vi "Choreo_Choreo_Globals.vi"() -> ()   [LabVIEW 2019, in "ChoreoLib.lvlib"]
doc: "Global variables for the Choreo Trajectory following system."
uses:
  ChoreoLib.lvlib
  TypeDef/ChoreoTrajectoryCacheSwerve.ctl
  TypeDef/ChoreoTrajectorySwerve.ctl
  TypeDef/ChoreoSwerveSample.ctl
  TypeDef/ChoreoEventMarker.ctl
  ENum/Choreo_Util_AllianceFlipType.ctl
panel:
  in  "AllianceFlipYearInfo":T2={"Year"=2026, "AllianceFlipType"=enum."ROTATE_AROUND", "FieldLength"=16.541, "FieldWidth"=8.0692}
  in  "TrajectoryCacheSwerve":T3
  # "NOTE: This will need to be updated\nevery year."
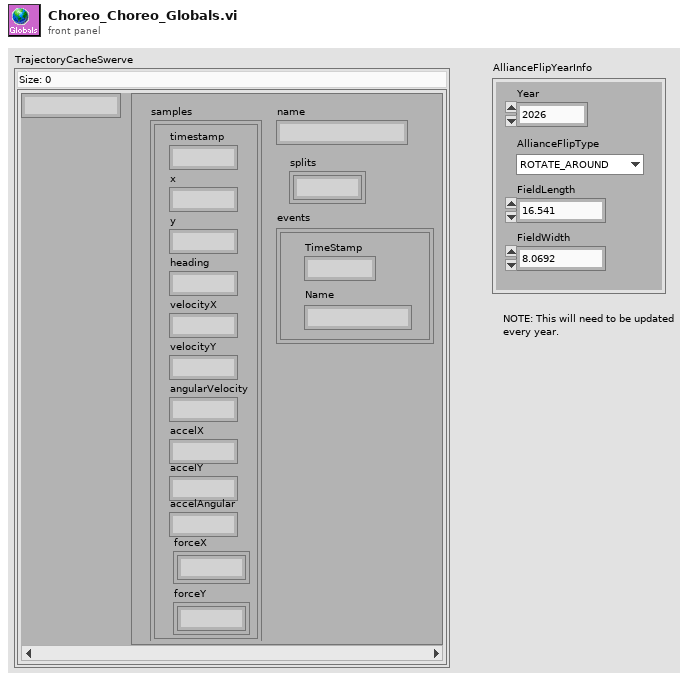
[diagram p1: front panel]
types:
  T1 = typedef "ChoreoLib.lvlib/Choreo_Util_AllianceFlipType.ctl" = enum16{"MIRRORED", "ROTATE_AROUND"}
  T2 = cluster{"Year":i32, "AllianceFlipType":T1, "FieldLength":dbl, "FieldWidth":dbl}
  T3 = typedef "ChoreoLib.lvlib/ChoreoTrajectoryCacheSwerve.ctl" = map{string, T4}
  T4 = typedef "ChoreoLib.lvlib/ChoreoTrajectorySwerve.ctl" = cluster{"name":string, "samples":T5[], "splits":i32[], "events":T6[]}
  T5 = typedef "ChoreoLib.lvlib/ChoreoSwerveSample.ctl" = cluster{"timestamp":dbl, "x":dbl, "y":dbl, "heading":dbl, "velocityX":dbl, "velocityY":dbl, "angularVelocity":dbl, "accelX":dbl, "accelY":dbl, "accelAngular":dbl, "forceX":dbl[], "forceY":dbl[]}
  T6 = typedef "ChoreoLib.lvlib/ChoreoEventMarker.ctl" = cluster{"TimeStamp":dbl, "Name":string}
diagram:
